vi "CfgManager Cache Lifetime Tests.vi"() -> ()   [LabVIEW 2013]
uses:
  Manager/ConfigManager.lvclass
  Manager/ConfigManager.lvclass/ConfigManager.ctl
  Serializer/Serializer.lvclass
  Encoding/Encoding.lvclass
  Encryption/Encryption.lvclass
  Collection/ConfigManagerCollection.lvclass
  Manager/Read Serializer.vi
  Manager/Read Encoding.vi
  Manager/Read Encryption.vi
  <vilib>/Utility/VariantDataType/GetTypeInfo.vi
  Manager/Decompose KVPs.vi
  <vilib>/LabVIEW Open Source/Data Manipulation/KVP Parser.vi
  Cache/ConfigManager.Cache.lvclass
panel:
  out "partial 2":variant
  out "partial 1":variant
  out "All Values":variant[](array[variant])
  out "All Keys":string[](array[string])
  out "Keys":string[](array[string])
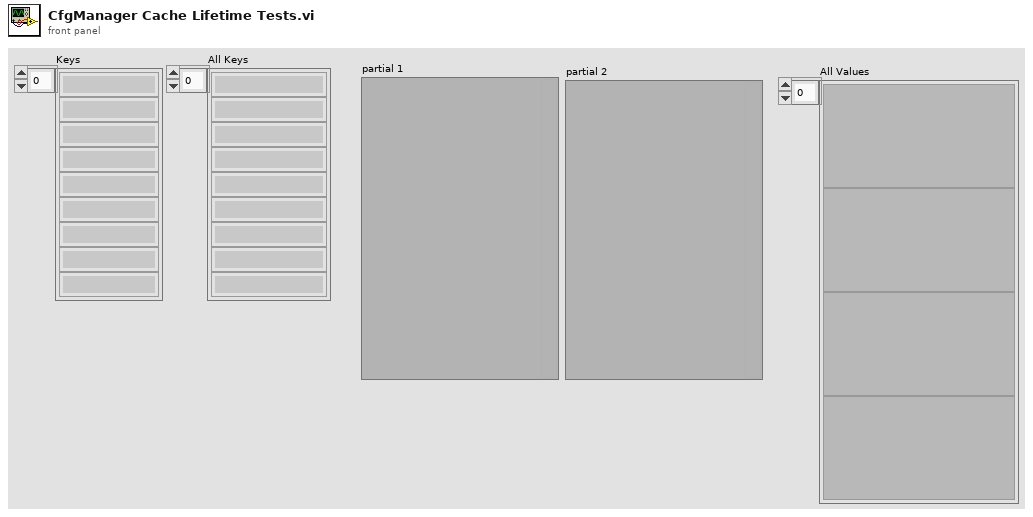
[diagram p1: front panel]
types:
  T1 = cluster{"status":bool, "code":i32, "source":string, "SubType":errorcluster}
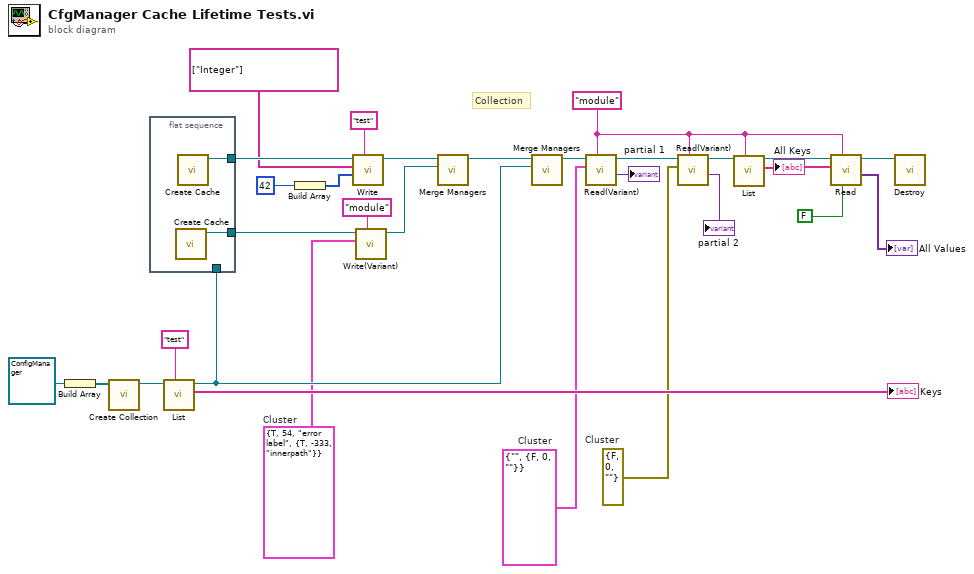
[diagram p0: block diagram]
diagram:
  w3 = errorcluster {"status"=FALSE, "code"=0, "source"=""}  # Cluster
  w7 = cluster{"source":string, "SubType":errorcluster} {"source"="", "SubType"={"status"=FALSE, "code"=0, "source"=""}}  # Cluster
  w9 = T1 {"status"=TRUE, "code"=54, "source"="error label", "SubType"={"status"=TRUE, "code"=-333, "source"="innerpath"}}  # Cluster
  w1 = "module" ("Qualified Name")
  # "Collection"
  n1 = Build Array(refnum<class "ConfigManager.lvclass"> refnum ("SMOConfig.lvlib:ConfigManager.lvclass")) -> (w27:refnum<class "ConfigManager.lvclass">[])
  n2 = call "Create Collection.vi"("List"=w27) -> ("SMOConfigManagerCollection out"=w26:refnum<class "ConfigManagerCollection.lvclass">)  [unwired: 10 in]
  n3 = flat-sequence {
    tunnel: [w32] -> w11
    tunnel: [w31] -> w29
    tunnel: w25 -> [_]
    frame #0 {
      n4 = call "Create Cache.vi"() -> ("ConfigManager.Cache"=w32:refnum<class "ConfigManager.Cache.lvclass">)  [unwired: 11 in]
      n5 = call "Create Cache.vi"() -> ("ConfigManager.Cache"=w31:refnum<class "ConfigManager.Cache.lvclass">)  [unwired: 11 in]
    }
  }
  n6 = call "List.vi"("Qualified Name"="test", "ConfigManager in"=w26) -> ("Keys"=→"Keys":string[], "ConfigManager out"=w25:refnum<class "ConfigManagerCollection.lvclass">)  [unwired: 7 in, 1 out]
  n7 = Build Array(42) -> (w16:i32[])
  n8 = call "Write.vi"("Qualified Name"="test", "Values"=w16, "keys"=string[] ["Integer"], "ConfigManager in"=w29) -> ("ConfigManager out"=w14:refnum<class "ConfigManager.Cache.lvclass">)  [unwired: 5 in, 2 out]
  n9 = call "Write(Variant).vi"("Qualified Name"="module", "value"=w9, "ConfigManager in"=w11) -> ("ConfigManager out"=w12:refnum<class "ConfigManager.Cache.lvclass">)  [unwired: 6 in, 2 out]
  n10 = call "Merge Managers.vi"("ConfigManager B"=w12, "ConfigManager A"=w14) -> ("ConfigManagerCollection"=w30:refnum<class "ConfigManagerCollection.lvclass">)  [unwired: 9 in]
  n11 = call "Merge Managers.vi"("ConfigManager B"=w25, "ConfigManager A"=w30) -> ("ConfigManagerCollection"=w8:refnum<class "ConfigManagerCollection.lvclass">)  [unwired: 9 in]
  n12 = call "Read(Variant).vi"("Qualified Name"=w1, "Type"=w7, "ConfigManager in"=w8) -> ("value"=→"partial 1":variant, "ConfigManager out"=w5:refnum<class "ConfigManagerCollection.lvclass">)  [unwired: 6 in, 1 out]
  n13 = call "Read(Variant).vi"("Qualified Name"=w1, "Type"=w3, "ConfigManager in"=w5) -> ("value"=→"partial 2":variant, "ConfigManager out"=w4:refnum<class "ConfigManagerCollection.lvclass">)  [unwired: 6 in, 1 out]
  n14 = call "List.vi"("Qualified Name"=w1, "ConfigManager in"=w4) -> ("Keys"=w18:string[], "ConfigManager out"=w20:refnum<class "ConfigManagerCollection.lvclass">)  [unwired: 7 in, 1 out]
  "All Keys" <- w18
  n15 = call "Read.vi"("prioritize Cache? (F)"=FALSE ("use Cache? (F)"), "Qualified Name"=w1, "keys in"=w18, "ConfigManager in"=w20) -> ("Values"=→"All Values":variant[], "ConfigManager out"=w19:refnum<class "ConfigManagerCollection.lvclass">)  [unwired: 4 in, 2 out]
  n16 = call-dynamic "Destroy.vi"("ConfigManagerCollection in"=w19) -> ()  [unwired: 9 in, 2 out]
